vi "XY Graph Cumulative Function.vi"(7 "Normalized (F)":bool, 8 "error in (no error)":errorcluster, 9 "Replace Plot (T)?":bool=TRUE, 11 "Selected Plot Info":T1={"Multiplot XY Graph"=refnum, "Mouse Coordinates"={"Horizontal"=0, "Vertical"=0}, "Plot Index"=-1}) -> (0 "Error Out":errorcluster, 1 "Cumulative Function Message":string, 3 "Cumulative Function":cluster{"t Array":dbl[], "IRF Array":dbl[]})   [LabVIEW 2021, in "XY Graph Add-Ons.lvlib"]
uses:
  XY Graph Add-Ons.lvlib
  XY Graph Selected Plot Info.ctl
  XY Graph Refnum.ctl
  <vilib>/Utility/miscctls.llb/LVPoint32TypeDef.ctl
  Arrays/Arrays.lvlib
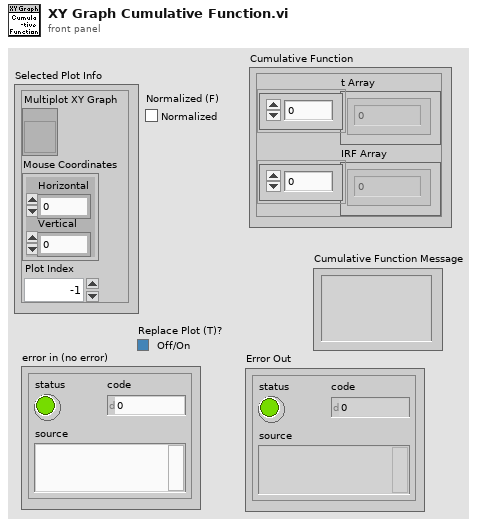
[diagram p1: front panel]
types:
  T1 = typedef "XY Graph Add-Ons.lvlib/XY Graph Selected Plot Info.ctl" = cluster{"Multiplot XY Graph":T2, "Mouse Coordinates":T3, "Plot Index":i32}
  T2 = typedef "XY Graph Add-Ons.lvlib/XY Graph Refnum.ctl" = refnum<vi>
  T3 = typedef "LVPoint32TypeDef.ctl" = cluster{"Horizontal":i32, "Vertical":i32}
  T4 = typedef "XY Graph Add-Ons.lvlib/XY Plot Data.ctl" = cluster{"X Array":dbl[], "Y Array":dbl[]}
  T5 = cluster{"X Array":dbl[], "Cumulative Function Array":dbl[]}
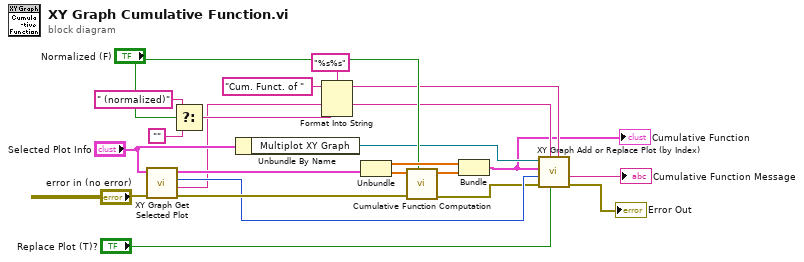
[diagram p0: block diagram]
diagram:
  n1 = call "XY Graph Get Selected Plot.vi"("error in (no error)"="error in (no error)", "Selected Plot Info"="Selected Plot Info") -> ("error out"=w11:errorcluster, "Plot Name"=w4:string, "Plot Index"=w8:i32, "Plot"=w15:T4)  [unwired: 4 in, 2 out]
  n2 = Select(t=" (normalized)" ("input 2"), s="Normalized (F)", f="") -> (s? t:f=w17:string)
  n3 = Unbundle By Name("Selected Plot Info") -> ("Multiplot XY Graph"=w9:T2)
  n4 = Format Into String(format string="%s%s", initial string="Cum. Funct. of ", w4, w17) -> (resulting string=w5:string)  [unwired: 1 in, 1 out]
  n5 = Unbundle(w15) -> ("X Array"=w12:dbl[], "Y Array"=w14:dbl[])
  n6 = call "Cumulative Function Computation.vi"("Normalized (F)"="Normalized (F)", "Error In"=w11, "Array"=w14) -> ("Error Out"=w7:errorcluster, "Cumulative Function Array"=w13:dbl[])  [unwired: 7 in]
  n7 = Bundle("X Array"=w12, "Cumulative Function Array"=w13) -> (w2:T5)  [unwired: 1 in]
  "Cumulative Function" <- w2
  n8 = call "XY Graph Add or Replace Plot (by Index).vi"("New Plot Name"=w5, "Replace Plot (T)?"="Replace Plot (T)?", "Original Plot Name"=w4, "error in (no error)"=w7, "Plot Index"=w8, "Plot in"=w2, "XYGraph in"=w9) -> ("error out"=→"Error Out":errorcluster, "Message"=→"Cumulative Function Message":string)  [unwired: 3 in]
